vi "Error Info.vi"(11 "error":T1) -> (2 "description":string, 3 "code":i32)   [LabVIEW 2017, in "DSF Core.lvlib" / "DSF PXImc Transceiver.lvclass"]
uses:
  DSF PXImc Transceiver.lvclass
  Errors.ctl
  Base Error Code.vi
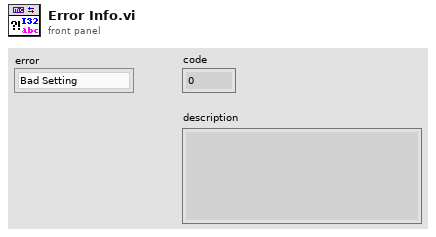
[diagram p1: front panel]
types:
  T1 = typedef "DSF Core.lvlib/DSF PXImc Transceiver.lvclass/Errors.ctl" = enum8{"Bad Setting", "Duplicate Stream ID"}
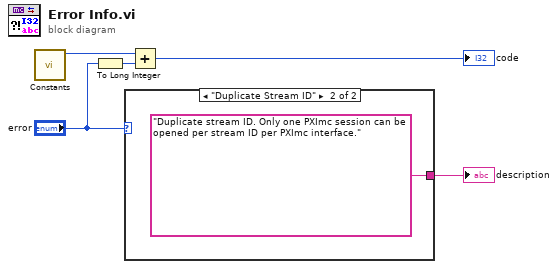
[diagram p0: block diagram]
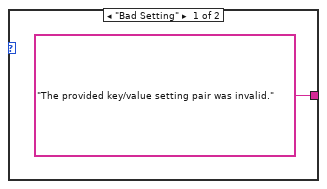
[diagram p2: hidden frame]
diagram:
  n1 = call-poly "Constants.vi"() -> ("pximc base error code"=w5:i32)  [unwired: 11 in]
  n2 = To Long Integer(number="error") -> (32bit integer=w4:i32)
  n3 = case shown="\"Duplicate Stream ID\"" "error" {
    tunnel: ["The provided key/value setting pair was invalid." "Duplicate stream ID. Only one PXImc session can be opened per stream ID per PXImc interface."] -> w1
    frame "Bad Setting" {
    }
    frame "Duplicate Stream ID" {
    }
  }
  "description" <- w1
  n4 = Add(x=w5, y=w4) -> (x+y=→"code":i32)
